vi "Agilent 6XXX Series Output Voltage.vi"(4 "time for output\nto stablize (5000 ms)":u32=5000, 6 "channel (1)":u8=1 min=1 max=4 step=1, 7 "delay (0 s)":dbl=0.5 min=0.0 max=32.767 format="%.3f", 8 "error in (no error)":errorcluster, 9 "current (0 A)":dbl=0.13 format="%.3f", 10 "voltage (0 V)":dbl format="%.3f", 11 "VISA resource name":refnum<visa-resource-name>) -> (0 "error out":errorcluster, 1 "output current":dbl format="%.4f", 2 "output voltage":dbl format="%.4f")   [LabVIEW 2020]
doc: "This Application Function sets the voltage, current and delay and reads back the output voltage and current using various subfunctions.\n\nNote: Before running this function, you must open the instrument session by running the Initialize function."
uses:
  <instrlib>/Agilent 6XXX Series/Agilent 6XXX Series.lvlib
panel:
  # "© 2005 National Instruments.  ALL RIGHTS RESERVED."
  # "*662xA only"
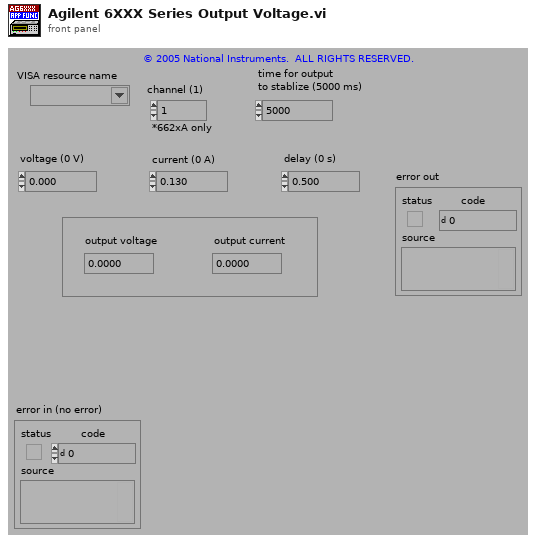
[diagram p1: front panel]
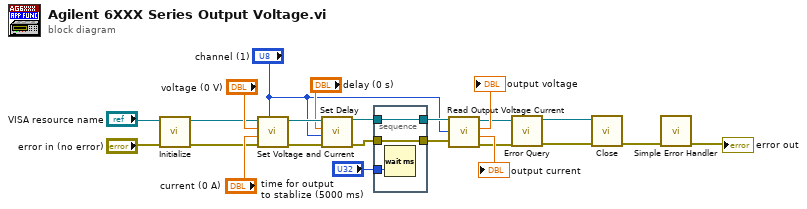
[diagram p0: block diagram]
diagram:
  n1 = call <instrlib>:"Initialize.vi"("error in (no error)"="error in (no error)", "VISA resource name"="VISA resource name") -> ("error out"=w6:errorcluster, "VISA resource name out"=w5:refnum<visa-resource-name>)  [unwired: 8 in]
  n2 = call <instrlib>:"Set Voltage and Current.vi"("channel (1)"="channel (1)", "error in (no error)"=w6, "current (0 A)"="current (0 A)", "voltage (0 V)"="voltage (0 V)", "VISA resource name"=w5) -> ("error out"=w20:errorcluster, "VISA resource name out"=w21:refnum<visa-resource-name>)  [unwired: 5 in]
  n3 = call <instrlib>:"Set Delay.vi"("error in (no error)"=w20, "channel (1)"="channel (1)", "delay (0 s)"="delay (0 s)", "VISA resource name"=w21) -> ("error out"=w14:errorcluster, "VISA resource name out"=w16:refnum<visa-resource-name>)  [unwired: 6 in]
  n4 = stacked-sequence {
    tunnel: w16 -> [w26]
    tunnel: [w26] -> w15
    tunnel: w14 -> [w25]
    tunnel: [w25] -> w13
    tunnel: "time for output\nto stablize (5000 ms)" -> [w24]
    frame #0 {
      n5 = Wait (ms)(milliseconds to wait=w24) -> ()  [unwired: 1 out]
    }
  }
  n6 = call <instrlib>:"Read Output Voltage Current.vi"("error in (no error)"=w13, "channel (1)"="channel (1)", "VISA resource name"=w15) -> ("error out"=w10:errorcluster, "output current"=→"output current":dbl, "output voltage"=→"output voltage":dbl, "VISA resource name out"=w11:refnum<visa-resource-name>)  [unwired: 5 in]
  n7 = call <instrlib>:"Error Query.vi"("error in (no error)"=w10, "VISA resource name"=w11) -> ("error out"=w3:errorcluster, "VISA resource name out"=w4:refnum<visa-resource-name>)  [unwired: 6 in, 2 out]
  n8 = call <instrlib>:"Close.vi"("error in (no error)"=w3, "VISA resource name"=w4) -> ("error out"=w2:errorcluster)  [unwired: 9 in]
  n9 = call <vilib>:"Simple Error Handler.vi"("error in (no error)"=w2) -> ("error out"=→"error out":errorcluster)  [unwired: 4 in, 4 out]
